vi "finalchannelselecthack_v2.vi"() -> (1 "devices":u32[](array[numeric]), 2 "Device chans":T1(array[cluster]))   [LabVIEW 2015]
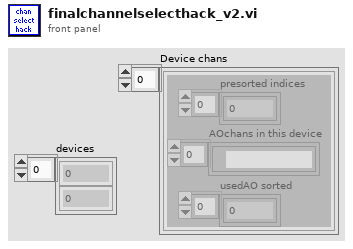
[diagram p1: front panel]
types:
  T1 = cluster{"presorted indices":i32[], "AOchans in this device":tag[], "usedAO sorted":i32[]}[]
  T2 = typedef "LVRectTypeDef.ctl" = cluster{"Left":i16, "Top":i16, "Right":i16, "Bottom":i16}
  T3 = cluster{"Xpixels":i32, "Vxminref":dbl, "Vxmaxref":dbl, "P":dbl, "Ypixels":i32, "Vyminref":dbl, "Vymaxref":dbl, "srate":sgl, "sAOxy":i32, "timeout":dbl, "type":string, "date":string, "time":string, "Colormap":u16, "Drawing Mode":u16, "Scanning Mode":u16, "square pixels":bool, "square matrix":bool, "Xpixels Img":i32, "Vx-min Img":dbl, "VX-max Img":dbl, "Ypixels Img":i32, "Vy-min Img":dbl, "Vy-max Img ":dbl, "Angle Img":dbl, "autoshutter":bool, "finite":bool, "cont":bool, "wavdet":bool, "measpoints":i32, "avpp":i32, "bufferAO":i32, "bufferAI":i32, "starttick":u32, "waveform":path, "Vx-ref":dbl, "Vy-ref":dbl, "refreshrate":dbl, "refreshbuffer":i32, "tt_cycles":i32, "motorref":refnum<k7>, "mirrorswitch":refnum<k7>, "sample mode":i32, "maxbufferAI":i32, "srateAODO":sgl, "bin":sgl, "Pel":sgl, "Angle draw":dbl, "srate Img":sgl, "ROIimg_plotbounds":T2, "auto OD":bool, "ODfilt":u16, "aAI":i32[], "aCI":i32[], "aAO":u32[], "aDO":u32[], "refwfsize":dbl, "Lifetime":bool, "Vz-Img":dbl, "Vz-ref":dbl, "Vz-reset":dbl, "AIoverride":bool, "aAS":u32[], "XYZstart":dbl[], "External 100KHz Clock?":bool}
  T4 = typedef "XYZStage.lvlib/XYZStage Configuration.ctl" = cluster{"VISA resource name":refnum<visa-resource-name>, "Timeout (3sec)":u32}
  T5 = cluster{"StageS":i32, "StageL":i32, "currmeas data dir":path, "image OD":u16, "contour OD":u16, "point OD":u16, "AOlines":tag[], "AIlines":tag[], "CI lines":tag[], "DO lines":tag[], "AO names":string[], "CI names":string[], "AI names":string[], "DO names":string[], "CIextensions":string[], "AIextensions":string[], "Voltage to Ygalvo":i32, "Voltage to Xgalvo":i32, "Voltage to patch":i32, "640 shutter":i32, "2P shutter":i32, "LT timestamp":u32, "Vp":i32, "Ip":i32, "camera trigger":i32, "master data dir":path, "voltage to Zpos":i32, "Vto2P":i32, "640 AO":i32, "488 AO":i32, "532 AO":i32, "640TTL":u32, "488TTL":u32, "532TTL":u32, "Device 1 sampleclock out":tag, "Device 1 Starttrigger out":tag, "Device 2 sampleclock in":tag, "Device 2 StartTrigger in ":tag, "2PODTTL":u32, "488 shutter":u32, "LCVR red":u32, "LCVR blue":u32, "Sutter Stage Config":T4, "Device 1 ext sampleclock in (100Khz)":tag}
  T6 = cluster{"presorted indices":i32[], "AOchans in this device":tag[], "usedAO sorted":i32[]}
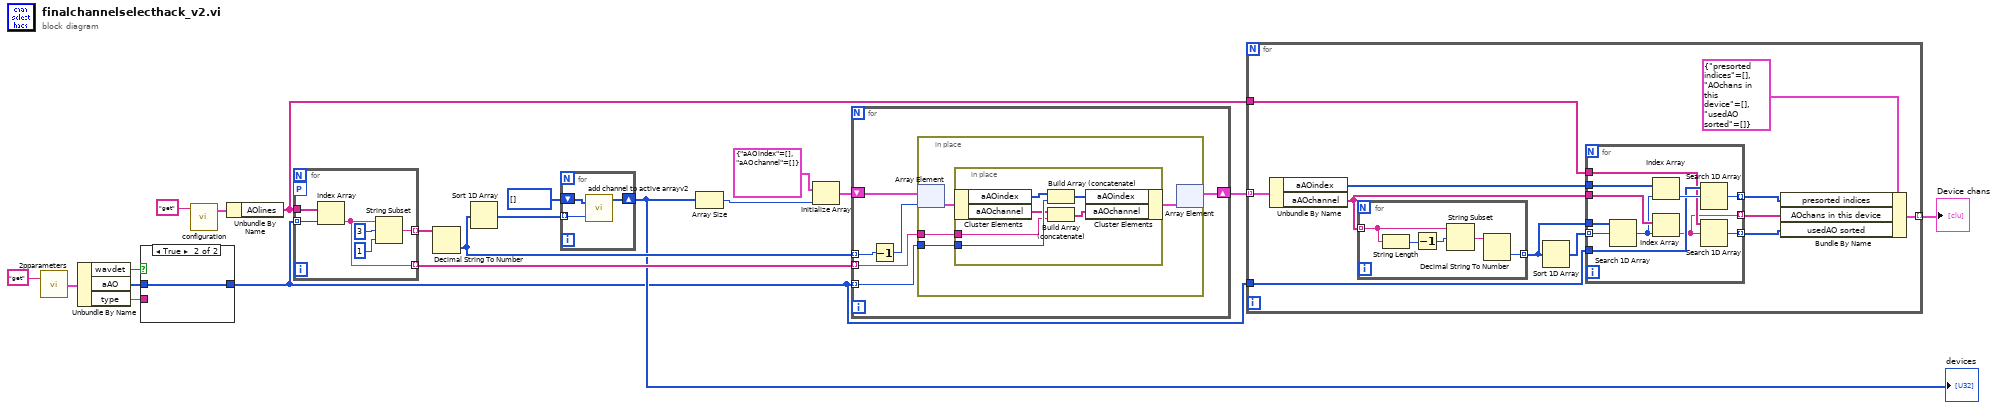
[diagram p0: block diagram]
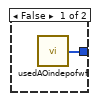
[diagram p2: hidden frame]
diagram:
  n1 = call "2pparameters.vi"("command"="get") -> ("params out"=w19:T3)  [unwired: 1 in]
  n2 = Unbundle By Name(w19) -> ("wavdet"=w17:bool, "aAO"=w18:u32[], "type"=w16:string)
  n3 = case shown="True" w17 {
    tunnel: w18 -> [_ w22]
    tunnel: [w21 w22] -> w3
    tunnel: w16 -> [_ _]
    frame False {
      n4 = call "usedAOindepofwf.vi"() -> ("AO"=w21:i32[])  [unwired: 1 in]
    }
    frame True {
    }
  }
  n5 = call "configuration.vi"("command"="get") -> ("config out"=w14:T5)  [unwired: 2 in, 1 out]
  n6 = Unbundle By Name(w14) -> ("AOlines"=w2:tag[])
  n7 = for {
    tunnel: w3 -> [w27] mode=indexing
    workers-P: _ -> [_]
    tunnel: w2 -> [w28]
    tunnel: [w26] -> w10 mode=indexing
    tunnel: [w23] -> w13 mode=indexing
    n8 = Index Array(array=w28, index=w27) -> (element=w26:tag)
    n9 = String Subset(string=w26, offset (0)=3, length (rest)=1 ("length (rest)")) -> (substring=w23:string)
  }
  n10 = Decimal String To Number(string=w13) -> (number=w9:i32[])  [unwired: 2 in, 1 out]
  n11 = Sort 1D Array(array=w9) -> (sorted array=w11:i32[])
  n12 = for {
    tunnel: w11 -> [w31] mode=indexing
    shift-right: [w29] -> w6
    shift-left: u32[] [] ("line array out") -> [w30]
    n13 = call "add channel to active arrayv2.vi"("line array in"=w30, "line to add"=w31) -> ("line array out"=w29:u32[])  [unwired: 2 out]
  }
  "devices" <- w6
  n14 = Array Size(array=w6) -> (size(s)=w7:i32)
  n15 = Initialize Array(cluster{"aAOindex":u32[], "aAOchannel":tag[]} {"aAOindex"=[], "aAOchannel"=[]} ("Cluster"), w7) -> (w5:cluster{"aAOindex":u32[], "aAOchannel":tag[]}[])
  n16 = for {
    tunnel: w10 -> [w32] mode=indexing
    tunnel: w9 -> [w37] mode=indexing
    tunnel: w3 -> [w33] mode=indexing
    shift-right: [w34] -> w4
    shift-left: w5 -> [w35]
    n17 = Decrement(x=w37) -> (x-1=w36:i32)
    n18 = in-place {
      in-place-border: w33 -> [w39]
      in-place-border: w32 -> [w38]
      n19 = in-place-array #1(w35, w36) -> (w41:cluster{"aAOindex":u32[], "aAOchannel":tag[]})
      n20 = in-place {
        in-place-border: w39 -> [w47]
        in-place-border: w38 -> [w46]
        n21 = in-place-cluster #2(w41) -> ("aAOindex"=w45:u32[], "aAOchannel"=w42:tag[])
        n22 = Build Array (concatenate)(w45, w47) -> (w44:u32[])
        n23 = Build Array (concatenate)(w42, w46) -> (w43:tag[])
        n24 = in-place-cluster #2("aAOindex"=w44, "aAOchannel"=w43) -> (w40:cluster{"aAOindex":u32[], "aAOchannel":tag[]})
      }
      n25 = in-place-array #1(w40) -> (w34:cluster{"aAOindex":u32[], "aAOchannel":tag[]}[])  [unwired: 1 out]
    }
  }
  n26 = for {
    tunnel: w4 -> [w59] mode=indexing
    tunnel: [w54] -> w1 mode=indexing
    tunnel: w3 -> [w52]
    tunnel: w2 -> [w49]
    n27 = Unbundle By Name(w59) -> ("aAOindex"=w53:u32[], "aAOchannel"=w56:tag[])
    n28 = for {
      tunnel: w56 -> [w71] mode=indexing
      tunnel: [w72] -> w57 mode=indexing
      n29 = String Length(string=w71) -> (length=w75:i32)
      n30 = Decrement(x=w75) -> (x-1=w74:i32)
      n31 = String Subset(string=w71, offset (0)=w74) -> (substring=w73:string)  [unwired: 1 in]
      n32 = Decimal String To Number(string=w73) -> (number=w72:i32)  [unwired: 2 in, 1 out]
    }
    n33 = Sort 1D Array(array=w57) -> (sorted array=w58:i32[])
    n34 = for {
      tunnel: w58 -> [w70] mode=indexing
      tunnel: w57 -> [w69]
      tunnel: w56 -> [w68]
      tunnel: [w61] -> w55 mode=indexing
      tunnel: w53 -> [w67]
      tunnel: w52 -> [w65]
      tunnel: [w64] -> w51 mode=indexing
      tunnel: w49 -> [w62]
      tunnel: [w60] -> w48 mode=indexing
      n35 = Search 1D Array(1D array=w69, element=w70) -> (index of element=w63:i32)  [unwired: 1 in]
      n36 = Index Array(array=w67, index=w63) -> (element=w66:u32)
      n37 = Index Array(array=w68, index=w63) -> (element=w61:tag)
      n38 = Search 1D Array(1D array=w65, element=w66) -> (index of element=w64:i32)  [unwired: 1 in]
      n39 = Search 1D Array(1D array=w62, element=w61) -> (index of element=w60:i32)  [unwired: 1 in]
    }
    n40 = Bundle By Name(cluster=T6 {"presorted indices"=[], "AOchans in this device"=[], "usedAO sorted"=[]}, "presorted indices"=w51, "AOchans in this device"=w55, "usedAO sorted"=w48) -> (w54:T6)
  }
  "Device chans" <- w1
